vi "UTILITY Read Config File.vi"(8 "Error In":errorcluster, 10 "Main Washer Display In":T1={"Appliance Details"={"FileVersionInfo"={"FileVersion"="", "ProductName"="", "InternalName"="", "CompanyName"="", "LegalCopyright"="", "FileDescription"=""}, "Dishwasher Info"={"Open Cup Weight (gm):"=0.0, "Auto Cup Weight (gm):"=0.0, "Detergent-Dish:"="", "Inlet Temperature-Dish:"="", "Cycle Mode-Dish:"="", "Unit Control-Dish:"="", "Manufacturer-Dish:"=""}, "Washer Info"={"Hot Water Temperature (Fahrenheit):"="", "Cold Water Temperature (Fahrenheit):"="", "Capacity (cu.ft):"=0.0, "Initial Cloth Weight:"=0.0, "Cloth Lot:"=0, "Model Family:"="", "Program Name:"="", "Cycle Selection:"="", "Wash Temperature:"="", "Rinse Temperature:"="", "Load Size:"=""}, "File Name Output Array"=[], "Calibration Output Array"=[], "Appliance Common"={"Engineer:"="", "Model Number:"="", "Serial Number:"="", "Comments:"="", "Station ID:"="", "Technician:"="", "TR Number:"="", "Lab ID:"="", "Voltage:"="", "Water Pressure (PSI):"="", "Test Date:"="", "Computer Name:"="", "IP Address:"="", "Ambient RH:"="", "Frequency:"="", "Build:"="", "Filename:"="", "Test Type:"="", "Load Run #:"=0, "Ambient Temperature (F):"="", "File Path:"=path "", "Cycles Per Year"=0}, "Water Heater"={"Heating Mode:"=""}, "Dryer"={"Heat Setting:"="", "Washer Water Temperature (60 ± 5°F):"=0, "Water Hardness (PPM):"=0, "Dryness Setting:"="", "Dryer Type:"="", "Exhaust:"="", "Drying Cycle:"="", "Load Type:"="", "Nominal Load Weight"="", "Dryer Initial IMC Data"={"Measured IMC (lbs)"=0.0, "Actual Initial RMC (%)"=0.0, "RMC (Desired %)"=0.0, "Bone Dry Wt(lbs)"=0.0, "Tolerance(%)"=0.0, "Actual Final RMC (%)"=0.0, "CEF (lbf/kWh)"=0.0, "Minimum Weight (lbf)"=0.0, "Average Weight (lbf)"=0.0, "Maximum Weight (lbf)"=0.0, "Measured IMC In Range?"=FALSE, "Moisture Reduction Factor"=55.5, "Field Use Factor"=1.04, "Empty Dryer Cold Weigth"=0.0, "Energy Standard"=enum."D2-Automatic Dryer", "Weight Cloth (lbs)"=0.0, "Relative Moisture Content (%)"=0.0, "Relative Moisture Content - Avg (%)"=0.0}}}, "Display Data (RLT)"={"Status Color"=0, "Serial Number Display"="", "Cycle Count Display"=0, "Station Label Display"="", "Current Run Start Time Display"=0.0, "Board ID Display"="", "RPM Display"=0, "Current Display"=0.0, "Current Path Display"=path "", "Saving Display"=FALSE, "Unit Type Display"=enum."", "Total Time On Display"=0.0, "UI Button"=FALSE}} {"Display Data (RLT)"."Current Display" format="%.2f"; "Display Data (RLT)"."Cycle Count Display" format="%04d"; "Appliance Details"."Dryer"."Dryer Initial IMC Data"."Maximum Weight (lbf)" format="%03_6g"; "Appliance Details"."Dryer"."Dryer Initial IMC Data"."Average Weight (lbf)" format="%03_6g"; "Appliance Details"."Dryer"."Dryer Initial IMC Data"."Minimum Weight (lbf)" format="%03_6g"; "Appliance Details"."Dryer"."Dryer Initial IMC Data"."CEF (lbf/kWh)" format="%03_6g"; "Appliance Details"."Dryer"."Dryer Initial IMC Data"."Actual Final RMC (%)" format="%03_6g"; "Appliance Details"."Dryer"."Dryer Initial IMC Data"."Tolerance(%)" format="%0#_6g"; "Appliance Details"."Dryer"."Dryer Initial IMC Data"."Bone Dry Wt(lbs)" format="%03_6g"; "Appliance Details"."Dryer"."Dryer Initial IMC Data"."RMC (Desired %)" format="%0#_6g"; "Appliance Details"."Dryer"."Dryer Initial IMC Data"."Actual Initial RMC (%)" format="%03_6g"; "Appliance Details"."Dryer"."Dryer Initial IMC Data"."Measured IMC (lbs)" format="%0#_6g"}, 11 "File Locations In":T10) -> (0 "Error Out":errorcluster, 1 "GEA Information Out":T12={"GEA Diagnostic Data - Washer"={"Speed (RPM)"=0, "Load Size"=0, "Temperature"=0, "Water Pressure"=0.0, "Detergent"=0, "Fabric Softener"=0, "Tub Direction"="", "Detergent Valve"=FALSE, "Fabric Softener Valve"=FALSE, "Recirculating Pump"=FALSE, "Drain Valve"=FALSE, "Hot Valve"=FALSE, "Cold Valve"=FALSE, "Lid Closed Status"="", "Lid Lock Status"="", "Error Count"=0, "IGBT Temperature (Deg C)"=0, "Motor Speed"=0, "Latched OOB"=0, "Raw OOB"=0, "Plaster Status"=0, "Inverter Power (W)"=0, "Target Speed(BRPM)"=0, "Latched Agitate Motor Temp (Deg C)"=0, "Current Motor Temp (Deg C)"=0, "Profiler Status"="", "Current Inverter Action"="", "Error Codes"="", "Lid Locked"=FALSE, "Lid Closed"=FALSE, "9E Diagnostic Data"={"Total Cycle Time (Min)"=0, "Total Cycle Count (Current)"=0, "Total Error Count"=0, "Machine Error History"=0, "Washer UI History"=0, "Inverter Error History"=0, "Cycle Storage Limit"=0, "Error Storage Limit"=0, "Cycle Pages Supported"=0, "Error Pages Supported"=0, "Inverter Reset Count"=0}, "9F Diagnostic Data"={"Cycle Buffer Index"="", "Page Number"="", "Total Cycle Count"=0, "Delay Start Time"=0, "Stain Selected"="", "Selected Cycle"=0, "eWash"="", "Soil Level"="", "Temperature"="", "Overnight Ready"="", "Spin Setting"="", "Control Lock Status"="", "Stain Remover"="", "Steam Assist"="", "My Cycle"="", "PreWash"="", "Debug Log Enabled"="", "Rinse"="", "Signal Level"="", "PreSoak"=""}}, "Software Version"={"Critical Major SW Version"="", "Critical Minor SW Version"="", "Major SW Version"="", "Minor SW Version"="", "Parametric Data Ver. Major"="", "Parametric Data Ver. Minor"="", "Diagnostics Data Ver. Major"="", "Diagnostics Data Ver. Minor"="", "Current Personality Setting"=""}, "Debug Search Parameters"={"Pause"=["MchStdby", "MchPz", "MchIdl", "Machine Standby", "Machine Pause", "Machine Idle"], "Run"=["MchRn", "Machine Run", "Resume Process"], "EOC"=["EOC"], "Error Codes"=["Error1", "try", "rty", "inverr"]}, "Message Count"=0, "Number of Messages"=0, "Partial Message String"="", "Full Message to Save"="", "Board ID"="", "Board Index"=0, "Source Address"=0, "Destination Address"=0, "Data to send"=[], "ReceivedData"=[], "Debug/GEA Data"=[], "Command"=0, "GEA2 Reference Out"=refnum, "GEA2 Event Registration"=refnum, "Bus Data"="", "GEA Data"=[], "Network Variable Location"=0, "Water Heater GEA2 Data"={"GEA2 Label Array"=[], "PID_PARAMETERS"=[], "SUPPORTED_MODES"=[], "Button Status"={"Switch 1"=FALSE, "Switch 2"=FALSE, "Switch 3"=FALSE, "Switch 4"=FALSE, "Switch 5"=FALSE, "Switch 6"=FALSE, "Switch 7"=FALSE, "Switch 8"=FALSE, "Switch 9"=FALSE, "Switch 10"=FALSE, "Switch 11"=FALSE, "Switch 12"=FALSE, "Switch 13"=FALSE, "Switch 14"=FALSE, "Switch 15"=FALSE, "Switch 16"=FALSE}, "Status Query"={"Days Remaining (For Std Electric and Vacation)"=0, "Unit Status"="", "Current Tank Temp in Deg F"=0, "Current Setpoint in Deg F"=0, "Filter Status (% used)"=0, "Fallback Status (Fallback heating mode)"="", "Fallback Temp"=0, "\"Set Mode\" Selection"=""}, "Service Error Codes"={"Reserved"=FALSE, "Reserved 1"=FALSE, "Reserved 2"=FALSE, "Reserved 3"=FALSE, "Reserved 4"=FALSE, "Reserved 5"=FALSE, "Reserved 6"=FALSE, "Reserved 7"=FALSE, "DataFlash Fail Status"=FALSE, "Stuck Key Fail Status"=FALSE, "Dry Tank Fail Status"=FALSE, "Miswire Fail Status"=FALSE, "Reserved 8"=FALSE, "Reserved 9"=FALSE, "Reserved 10"=FALSE, "Reserved 11"=FALSE, "UE Fail Status"=FALSE, "LE Fail Status"=FALSE, "Filter Fail Status"=FALSE, "T3A Fail Status"=FALSE, "T3B Fail Status"=FALSE, "T4 Fail Status"=FALSE, "T5 Fail Status"=FALSE, "T2 Fail Status"=FALSE, "SS Cond A Status"=FALSE, "SS Cond B Status"=FALSE, "SS Cond C Status"=FALSE, "SS Cond D Status"=FALSE, "SS Cond E Status"=FALSE, "SS Cond F Status"=FALSE, "SS Fan Status"=FALSE, "CMP Fail Status"=FALSE}, "HEM_KWH_DATA"=[], "OTHER_FAULT_COUNTS"=[], "GEA2 Raw Message"="", "Hyperterminal Data"={"Source"=0, "Destination"=0, "Command"=0, "Length"=0, "CRC"=0, "UE - state (1/0 on off)"=0, "LE - state (1/0 on off)"=0, "Comp - state (1/0 on off)"=0, "Fan  - state (1/0 on off)"=0, "Setpoint Deg F"=0, "T2(TankSensor)"=0.0, "T3A(EvapIn)"=0.0, "T3B(EvapOut)"=0.0, "T4(CompressorDischarge)"=0.0, "T5(Ambient)"=0.0, "Current"=0.0, "Voltage (Volts)"=0, "EEV Position (0-480)"=0, "Reason for last heating cycle termination"=0, "Reason Data word 1"="", "Reason Data word 2"="", "Reason Data word 3"="", "Reason Data word 4"="", "SW Debug Data"="", "Flow Events (Bit Encoded)"=0, "Heating Control Mode"=0}, "Extra Data"={"Water Capacity (Gallons)"=0, "Max Vacation Duration Days"=0, "Min Vacation Duration Days"=0, "Max Set Point (Deg F)"=0, "Min Set Point (Deg F)"=0, "T5 Resistance"=0, "T4 Resistance"=0, "T3B Resistance"=0, "T2 Resistance"=0, "STD_ELEC_RANGE"="", "SS_FAULT_COUNTS"="", "SERIAL_NUMBER"="", "READ_PERSONALITY"=0, "RQST_OVERRIDE_STATUS"="", "MODEL_SELECT_AD_VALUE"=0, "MODEL NUMBER"="", "IDLB_RESISTANCE"=0, "DSM Override Status"="", "RQST_DATA_FROM_Memory"="", "RQST_DATA_FROM_DATA_FLASH"="", "RQST_CURRENT_PID_SH_TARGET"=0, "Unit System Mode"=""}}} {"Water Heater GEA2 Data"."Hyperterminal Data"."CRC" format="%x"; "Water Heater GEA2 Data"."Hyperterminal Data"."Length" format="%x"; "Water Heater GEA2 Data"."Hyperterminal Data"."Command" format="%x"; "Water Heater GEA2 Data"."Hyperterminal Data"."Destination" format="%x"; "Water Heater GEA2 Data"."Hyperterminal Data"."Source" format="%x"; "Destination Address" format="%x"; "Source Address" format="%x"; "Command" format="%.0x"; "Data to send" format="%x"; "ReceivedData" format="%x"}, 2 "Main Washer Display Out":T1={"Appliance Details"={"FileVersionInfo"={"FileVersion"="", "ProductName"="", "InternalName"="", "CompanyName"="", "LegalCopyright"="", "FileDescription"=""}, "Dishwasher Info"={"Open Cup Weight (gm):"=0.0, "Auto Cup Weight (gm):"=0.0, "Detergent-Dish:"="", "Inlet Temperature-Dish:"="", "Cycle Mode-Dish:"="", "Unit Control-Dish:"="", "Manufacturer-Dish:"=""}, "Washer Info"={"Hot Water Temperature (Fahrenheit):"="", "Cold Water Temperature (Fahrenheit):"="", "Capacity (cu.ft):"=0.0, "Initial Cloth Weight:"=0.0, "Cloth Lot:"=0, "Model Family:"="", "Program Name:"="", "Cycle Selection:"="", "Wash Temperature:"="", "Rinse Temperature:"="", "Load Size:"=""}, "File Name Output Array"=[], "Calibration Output Array"=[], "Appliance Common"={"Engineer:"="", "Model Number:"="", "Serial Number:"="", "Comments:"="", "Station ID:"="", "Technician:"="", "TR Number:"="", "Lab ID:"="", "Voltage:"="", "Water Pressure (PSI):"="", "Test Date:"="", "Computer Name:"="", "IP Address:"="", "Ambient RH:"="", "Frequency:"="", "Build:"="", "Filename:"="", "Test Type:"="", "Load Run #:"=0, "Ambient Temperature (F):"="", "File Path:"=path "", "Cycles Per Year"=60}, "Water Heater"={"Heating Mode:"=""}, "Dryer"={"Heat Setting:"="", "Washer Water Temperature (60 ± 5°F):"=60, "Water Hardness (PPM):"=17, "Dryness Setting:"="", "Dryer Type:"="", "Exhaust:"="", "Drying Cycle:"="", "Load Type:"="", "Nominal Load Weight"="", "Dryer Initial IMC Data"={"Measured IMC (lbs)"=7.0, "Actual Initial RMC (%)"=7.0, "RMC (Desired %)"=100.0, "Bone Dry Wt(lbs)"=7.0, "Tolerance(%)"=5.0, "Actual Final RMC (%)"=0.0, "CEF (lbf/kWh)"=0.0, "Minimum Weight (lbf)"=0.0, "Average Weight (lbf)"=0.0, "Maximum Weight (lbf)"=0.0, "Measured IMC In Range?"=FALSE, "Moisture Reduction Factor"=55.5, "Field Use Factor"=1.04, "Empty Dryer Cold Weigth"=0.0, "Energy Standard"=enum."D2-Automatic Dryer", "Weight Cloth (lbs)"=0.0, "Relative Moisture Content (%)"=0.0, "Relative Moisture Content - Avg (%)"=0.0}}}, "Display Data (RLT)"={"Status Color"=0, "Serial Number Display"="", "Cycle Count Display"=0, "Station Label Display"="", "Current Run Start Time Display"=0.0, "Board ID Display"="", "RPM Display"=0, "Current Display"=0.0, "Current Path Display"=path "", "Saving Display"=FALSE, "Unit Type Display"=enum."", "Total Time On Display"=0.0, "UI Button"=FALSE}} {"Display Data (RLT)"."Current Display" format="%.2f"; "Display Data (RLT)"."Cycle Count Display" format="%04d"; "Appliance Details"."Dryer"."Dryer Initial IMC Data"."Maximum Weight (lbf)" format="%03_6g"; "Appliance Details"."Dryer"."Dryer Initial IMC Data"."Average Weight (lbf)" format="%03_6g"; "Appliance Details"."Dryer"."Dryer Initial IMC Data"."Minimum Weight (lbf)" format="%03_6g"; "Appliance Details"."Dryer"."Dryer Initial IMC Data"."CEF (lbf/kWh)" format="%03_6g"; "Appliance Details"."Dryer"."Dryer Initial IMC Data"."Actual Final RMC (%)" format="%03_6g"; "Appliance Details"."Dryer"."Dryer Initial IMC Data"."Tolerance(%)" format="%0#_6g"; "Appliance Details"."Dryer"."Dryer Initial IMC Data"."Bone Dry Wt(lbs)" format="%03_6g"; "Appliance Details"."Dryer"."Dryer Initial IMC Data"."RMC (Desired %)" format="%0#_6g"; "Appliance Details"."Dryer"."Dryer Initial IMC Data"."Actual Initial RMC (%)" format="%03_6g"; "Appliance Details"."Dryer"."Dryer Initial IMC Data"."Measured IMC (lbs)" format="%0#_6g"})   [LabVIEW 2018]
uses:
  Washer HCC/Washer HCC NEWFI/Type Definitions/ViperHawk/ViperHawk Data.ctl
  Washer HCC/Washer HCC NEWFI/Type Definitions/ViperHawk/ViperHawk Diagnostic Data.ctl
  Save File/Public/Type Definitions/Save File Software Version.ctl
  Washer HCC/Washer HCC NEWFI/Type Definitions/ViperHawk/ViperHawk Search Control.ctl
  C:/Andrew_Treasure_Chest/NI-2010/Trunk/Utility/LabVIEW GEA2 Toolkit v1.0.0.0/Appliance.NET/GeaCommunication.dll
  LabVIEW GEA2 Toolkit v1.0.0.0/Appliance.NET/GeaCommunication.dll
  LabVIEW GEA2 Toolkit v1.0.0.0/type defs/Data Out.ctl
  GEA2 Commands/HEWH/Type Definitions/GEA2 Commands WaterHeater GEA2 Data.ctl
  GEA2 Commands/HEWH/Type Definitions/GEA2 Commands Button Status.ctl
  GEA2 Commands/HEWH/Type Definitions/GEA2 Commands Status Query.ctl
  GEA2 Commands/HEWH/Type Definitions/GEA2 Commands Service Error Codes.ctl
  Save File/Public/Type Definitions/Save File Washer.ctl
  Save File/File Setup (Public)/Type Definition/Save File DISH Dishwasher Details.ctl
  <vilib>/Platform/fileVersionInfo.llb/FileVersionInformation.ctl
  Washer DOE/Type Definitions/DOE Appliance Common.ctl
  Custom Pallet Controls/Custom Pallet String.ctl
  Save File/File Setup (Public)/Type Definition/DPT IMC Data.ctl
  Washer DOE/Type Definitions/DOE Dryer Standard.ctl
  Save File/Public/Type Definitions/Save File Appliance Display.ctl
  Save File/Public/Type Definitions/Save File Unit Type.ctl
  Save File/File Setup (Public)/Type Definition/Save File DOE File Path Control.ctl
  Save File/File Setup (Public)/Type Definition/Save File DOE Data Save Filepaths.ctl
  LabVIEW GEA2 Toolkit v1.0.0.0/library/GEA2_Toolkit.lvlib
  Save File/Save File.lvlib
  Save File/File Setup.lvlib
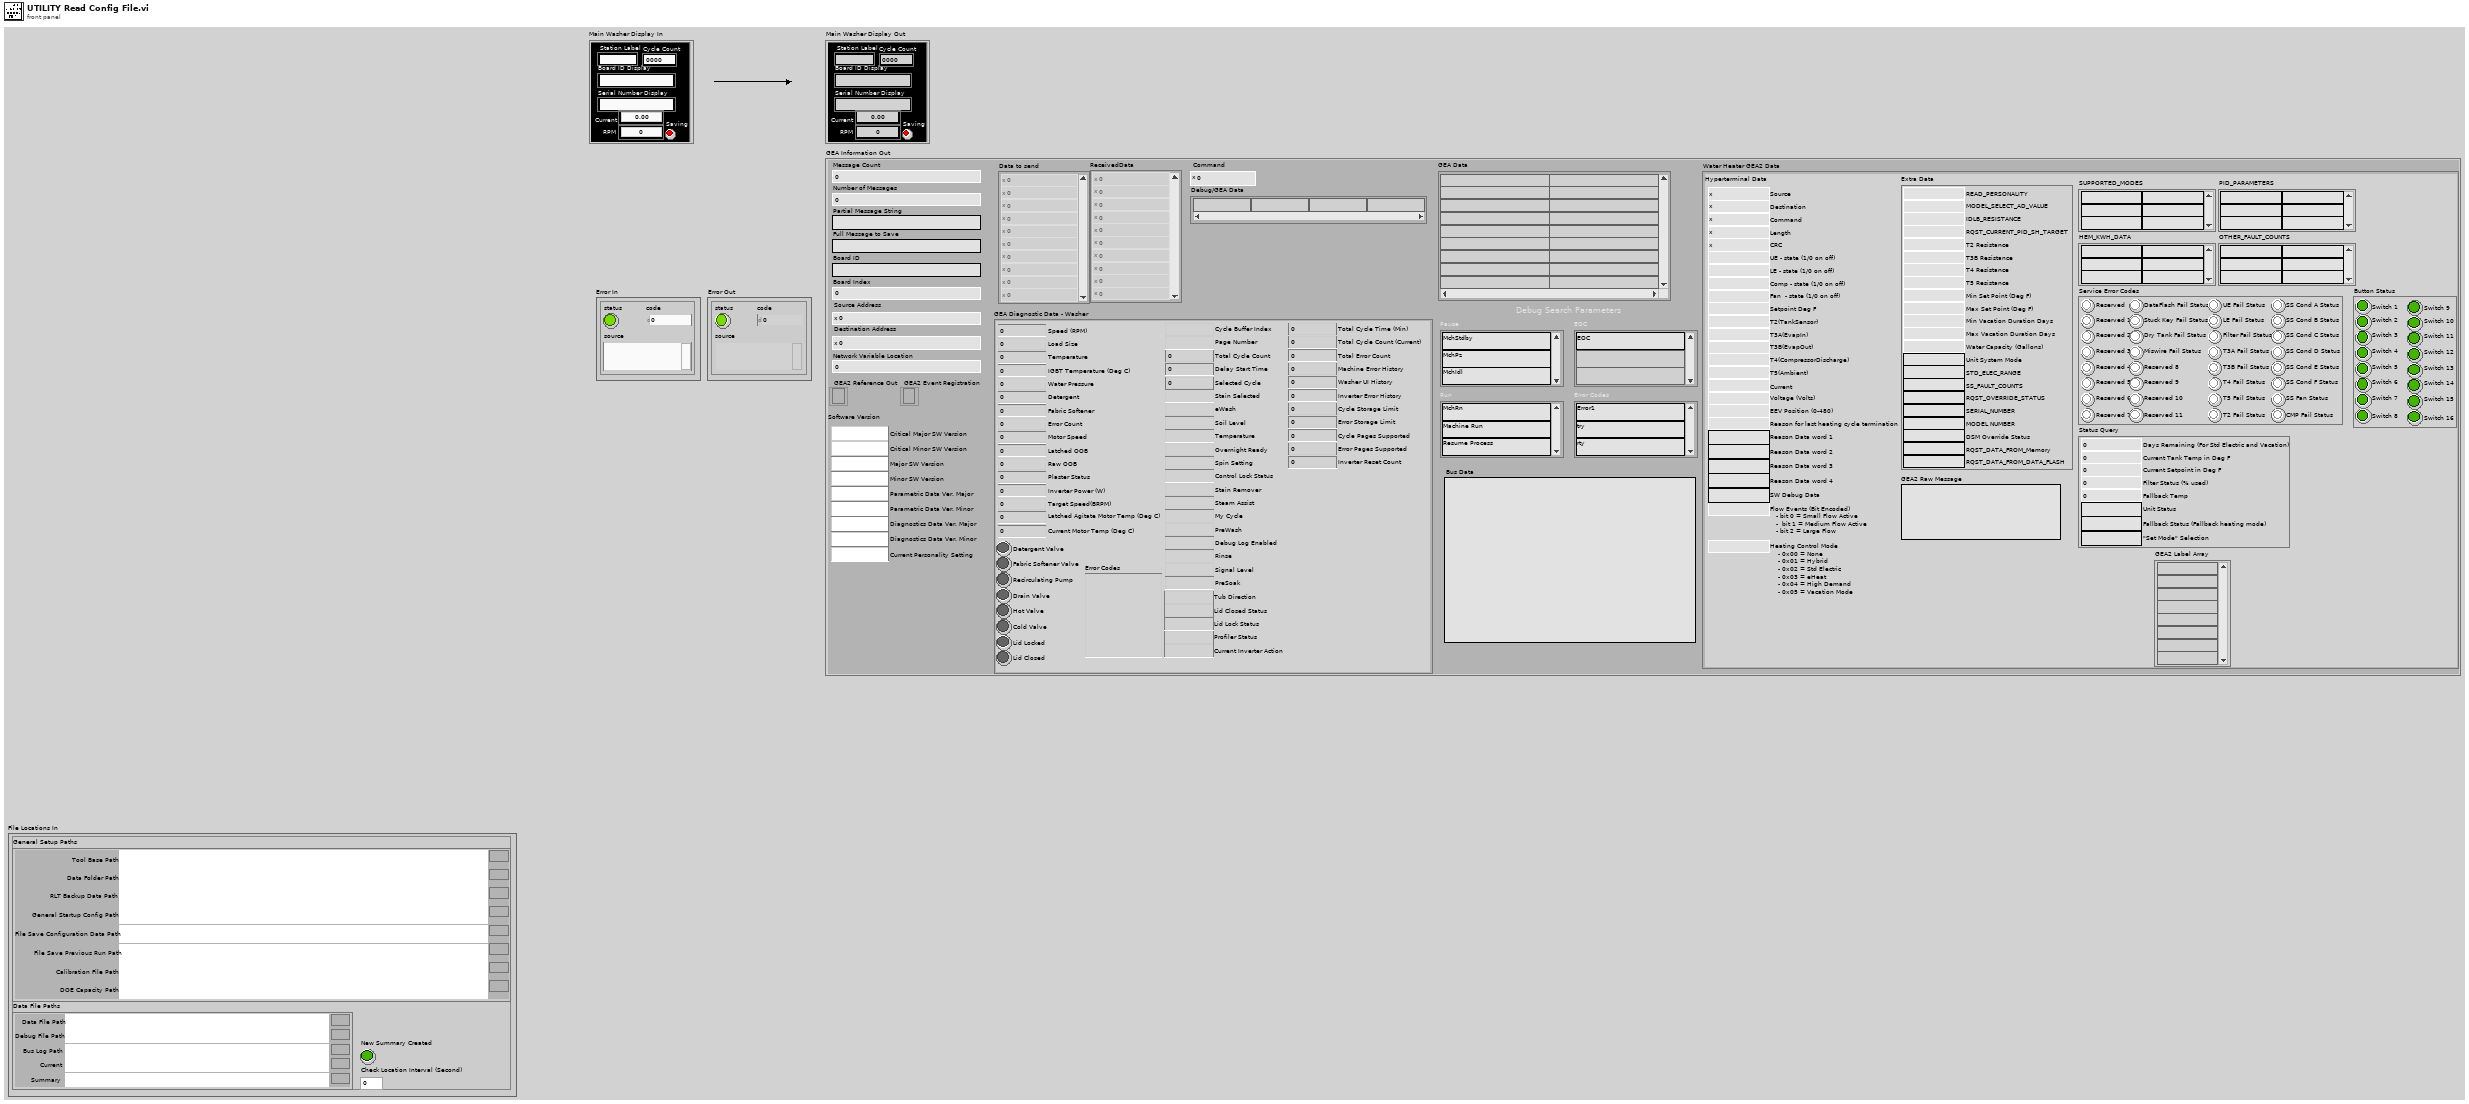
[diagram p1: front panel]
types:
  T1 = typedef "Save File.lvlib/Save File Washer.ctl" = cluster{"Appliance Details":T2, "Display Data (RLT)":T8}
  T2 = typedef "File Setup.lvlib/Save File DISH Dishwasher Details.ctl" = cluster{"FileVersionInfo":T3, "Dishwasher Info":cluster{"Open Cup Weight (gm):":dbl, "Auto Cup Weight (gm):":dbl, "Detergent-Dish:":string, "Inlet Temperature-Dish:":string, "Cycle Mode-Dish:":string, "Unit Control-Dish:":string, "Manufacturer-Dish:":string}, "Washer Info":cluster{"Hot Water Temperature (Fahrenheit):":string, "Cold Water Temperature (Fahrenheit):":string, "Capacity (cu.ft):":dbl, "Initial Cloth Weight:":dbl, "Cloth Lot:":i32, "Model Family:":string, "Program Name:":string, "Cycle Selection:":string, "Wash Temperature:":string, "Rinse Temperature:":string, "Load Size:":string}, "File Name Output Array":string[][], "Calibration Output Array":string[][], "Appliance Common":T4, "Water Heater":cluster{"Heating Mode:":string}, "Dryer":cluster{"Heat Setting:":T5, "Washer Water Temperature (60 ± 5°F):":u16, "Water Hardness (PPM):":u16, "Dryness Setting:":T5, "Dryer Type:":string, "Exhaust:":string, "Drying Cycle:":string, "Load Type:":string, "Nominal Load Weight":string, "Dryer Initial IMC Data":T6}}
  T3 = typedef "FileVersionInformation.ctl" = cluster{"FileVersion":string, "ProductName":string, "InternalName":string, "CompanyName":string, "LegalCopyright":string, "FileDescription":string}
  T4 = typedef "DOE Appliance Common.ctl" = cluster{"Engineer:":string, "Model Number:":string, "Serial Number:":string, "Comments:":string, "Station ID:":string, "Technician:":string, "TR Number:":string, "Lab ID:":string, "Voltage:":string, "Water Pressure (PSI):":string, "Test Date:":string, "Computer Name:":string, "IP Address:":string, "Ambient RH:":string, "Frequency:":string, "Build:":string, "Filename:":string, "Test Type:":string, "Load Run #:":i32, "Ambient Temperature (F):":string, "File Path:":path, "Cycles Per Year":u32}
  T5 = typedef "Custom Pallet String.ctl" = string
  T6 = typedef "DPT IMC Data.ctl" = cluster{"Measured IMC (lbs)":dbl, "Actual Initial RMC (%)":dbl, "RMC (Desired %)":dbl, "Bone Dry Wt(lbs)":dbl, "Tolerance(%)":dbl, "Actual Final RMC (%)":dbl, "CEF (lbf/kWh)":dbl, "Minimum Weight (lbf)":dbl, "Average Weight (lbf)":dbl, "Maximum Weight (lbf)":dbl, "Measured IMC In Range?":bool, "Moisture Reduction Factor":dbl, "Field Use Factor":dbl, "Empty Dryer Cold Weigth":dbl, "Energy Standard":T7, "Weight Cloth (lbs)":dbl, "Relative Moisture Content (%)":dbl, "Relative Moisture Content - Avg (%)":dbl}
  T7 = typedef "DOE Dryer Standard.ctl" = enum16{"D2-Automatic Dryer", "D2-Timer Dryer", "D1-Automatic Dryer", "D1-Timer Dryer", "Other"}
  T8 = typedef "Save File Appliance Display.ctl" = cluster{"Status Color":u32, "Serial Number Display":string, "Cycle Count Display":i32, "Station Label Display":string, "Current Run Start Time Display":dbl, "Board ID Display":string, "RPM Display":u32, "Current Display":dbl, "Current Path Display":path, "Saving Display":bool, "Unit Type Display":T9, "Total Time On Display":dbl, "UI Button":bool}
  T9 = typedef "Save File.lvlib/Save File Unit Type.ctl" = enum32{"", "Viper", "Hawk", "2015"}
  T10 = typedef "File Setup.lvlib/Save File DOE File Path Control.ctl" = cluster{"General Setup Paths":cluster{"Calibration File Path":path, "DOE Capacity Path":path, "Data Folder Path":path, "RLT Backup Data Path":path, "Tool Base Path":path, "General Startup Config Path":path, "File Save Previous Run Path":path, "File Save Configuration Data Path":path}, "Data File Paths":T11, "New Summary Created":bool, "Check Location Interval (Second)":i32}
  T11 = typedef "File Setup.lvlib/Save File DOE Data Save Filepaths.ctl" = cluster{"Data File Path":path, "Debug File Path":path, "Bus Log Path":path, "Current":path, "Summary":path}
  T12 = typedef "ViperHawk Data.ctl" = cluster{"GEA Diagnostic Data - Washer":T13, "Software Version":T14, "Debug Search Parameters":T15, "Message Count":i32, "Number of Messages":i32, "Partial Message String":string, "Full Message to Save":string, "Board ID":string, "Board Index":i32, "Source Address":u8, "Destination Address":u8, "Data to send":u8[], "ReceivedData":u8[], "Debug/GEA Data":string[], "Command":u8, "GEA2 Reference Out":refnum<k24>, "GEA2 Event Registration":refnum<event-registration>, "Bus Data":string, "GEA Data":string[][], "Network Variable Location":i32, "Water Heater GEA2 Data":T16}
  T13 = typedef "ViperHawk Diagnostic Data.ctl" = cluster{"Speed (RPM)":u32, "Load Size":u32, "Temperature":u32, "Water Pressure":dbl, "Detergent":u32, "Fabric Softener":u32, "Tub Direction":string, "Detergent Valve":bool, "Fabric Softener Valve":bool, "Recirculating Pump":bool, "Drain Valve":bool, "Hot Valve":bool, "Cold Valve":bool, "Lid Closed Status":string, "Lid Lock Status":string, "Error Count":u32, "IGBT Temperature (Deg C)":u32, "Motor Speed":u32, "Latched OOB":u32, "Raw OOB":u32, "Plaster Status":u32, "Inverter Power (W)":u32, "Target Speed(BRPM)":u32, "Latched Agitate Motor Temp (Deg C)":u32, "Current Motor Temp (Deg C)":u32, "Profiler Status":string, "Current Inverter Action":string, "Error Codes":string, "Lid Locked":bool, "Lid Closed":bool, "9E Diagnostic Data":cluster{"Total Cycle Time (Min)":u32, "Total Cycle Count (Current)":u16, "Total Error Count":u16, "Machine Error History":u32, "Washer UI History":u32, "Inverter Error History":u32, "Cycle Storage Limit":u8, "Error Storage Limit":u8, "Cycle Pages Supported":u8, "Error Pages Supported":u8, "Inverter Reset Count":u16}, "9F Diagnostic Data":cluster{"Cycle Buffer Index":string, "Page Number":string, "Total Cycle Count":u32, "Delay Start Time":u32, "Stain Selected":string, "Selected Cycle":u32, "eWash":string, "Soil Level":string, "Temperature":string, "Overnight Ready":string, "Spin Setting":string, "Control Lock Status":string, "Stain Remover":string, "Steam Assist":string, "My Cycle":string, "PreWash":string, "Debug Log Enabled":string, "Rinse":string, "Signal Level":string, "PreSoak":string}}
  T14 = typedef "Save File.lvlib/Save File Software Version.ctl" = cluster{"Critical Major SW Version":string, "Critical Minor SW Version":string, "Major SW Version":string, "Minor SW Version":string, "Parametric Data Ver. Major":string, "Parametric Data Ver. Minor":string, "Diagnostics Data Ver. Major":string, "Diagnostics Data Ver. Minor":string, "Current Personality Setting":string}
  T15 = typedef "ViperHawk Search Control.ctl" = cluster{"Pause":string[], "Run":string[], "EOC":string[], "Error Codes":string[]}
  T16 = typedef "GEA2 Commands WaterHeater GEA2 Data.ctl" = cluster{"GEA2 Label Array":string[], "PID_PARAMETERS":string[][], "SUPPORTED_MODES":string[][], "Button Status":T17, "Status Query":T18, "Service Error Codes":T19, "HEM_KWH_DATA":string[][], "OTHER_FAULT_COUNTS":string[][], "GEA2 Raw Message":string, "Hyperterminal Data":cluster{"Source":u8, "Destination":u8, "Command":u8, "Length":u8, "CRC":u16, "UE - state (1/0 on off)":u8, "LE - state (1/0 on off)":u8, "Comp - state (1/0 on off)":u8, "Fan  - state (1/0 on off)":u8, "Setpoint Deg F":i32, "T2(TankSensor)":dbl, "T3A(EvapIn)":dbl, "T3B(EvapOut)":dbl, "T4(CompressorDischarge)":dbl, "T5(Ambient)":dbl, "Current":dbl, "Voltage (Volts)":u16, "EEV Position (0-480)":u16, "Reason for last heating cycle termination":u16, "Reason Data word 1":string, "Reason Data word 2":string, "Reason Data word 3":string, "Reason Data word 4":string, "SW Debug Data":string, "Flow Events (Bit Encoded)":u16, "Heating Control Mode":u16}, "Extra Data":cluster{"Water Capacity (Gallons)":u32, "Max Vacation Duration Days":u32, "Min Vacation Duration Days":u32, "Max Set Point (Deg F)":u32, "Min Set Point (Deg F)":u32, "T5 Resistance":u32, "T4 Resistance":u32, "T3B Resistance":u32, "T2 Resistance":u32, "STD_ELEC_RANGE":string, "SS_FAULT_COUNTS":string, "SERIAL_NUMBER":string, "READ_PERSONALITY":u8, "RQST_OVERRIDE_STATUS":string, "MODEL_SELECT_AD_VALUE":u32, "MODEL NUMBER":string, "IDLB_RESISTANCE":u32, "DSM Override Status":string, "RQST_DATA_FROM_Memory":string, "RQST_DATA_FROM_DATA_FLASH":string, "RQST_CURRENT_PID_SH_TARGET":u16, "Unit System Mode":string}}
  T17 = typedef "GEA2 Commands Button Status.ctl" = cluster{"Switch 1":bool, "Switch 2":bool, "Switch 3":bool, "Switch 4":bool, "Switch 5":bool, "Switch 6":bool, "Switch 7":bool, "Switch 8":bool, "Switch 9":bool, "Switch 10":bool, "Switch 11":bool, "Switch 12":bool, "Switch 13":bool, "Switch 14":bool, "Switch 15":bool, "Switch 16":bool}
  T18 = typedef "GEA2 Commands Status Query.ctl" = cluster{"Days Remaining (For Std Electric and Vacation)":u8, "Unit Status":string, "Current Tank Temp in Deg F":u8, "Current Setpoint in Deg F":u8, "Filter Status (% used)":u8, "Fallback Status (Fallback heating mode)":string, "Fallback Temp":u8, "\"Set Mode\" Selection":string}
  T19 = typedef "GEA2 Commands Service Error Codes.ctl" = cluster{"Reserved":bool, "Reserved 1":bool, "Reserved 2":bool, "Reserved 3":bool, "Reserved 4":bool, "Reserved 5":bool, "Reserved 6":bool, "Reserved 7":bool, "DataFlash Fail Status":bool, "Stuck Key Fail Status":bool, "Dry Tank Fail Status":bool, "Miswire Fail Status":bool, "Reserved 8":bool, "Reserved 9":bool, "Reserved 10":bool, "Reserved 11":bool, "UE Fail Status":bool, "LE Fail Status":bool, "Filter Fail Status":bool, "T3A Fail Status":bool, "T3B Fail Status":bool, "T4 Fail Status":bool, "T5 Fail Status":bool, "T2 Fail Status":bool, "SS Cond A Status":bool, "SS Cond B Status":bool, "SS Cond C Status":bool, "SS Cond D Status":bool, "SS Cond E Status":bool, "SS Cond F Status":bool, "SS Fan Status":bool, "CMP Fail Status":bool}
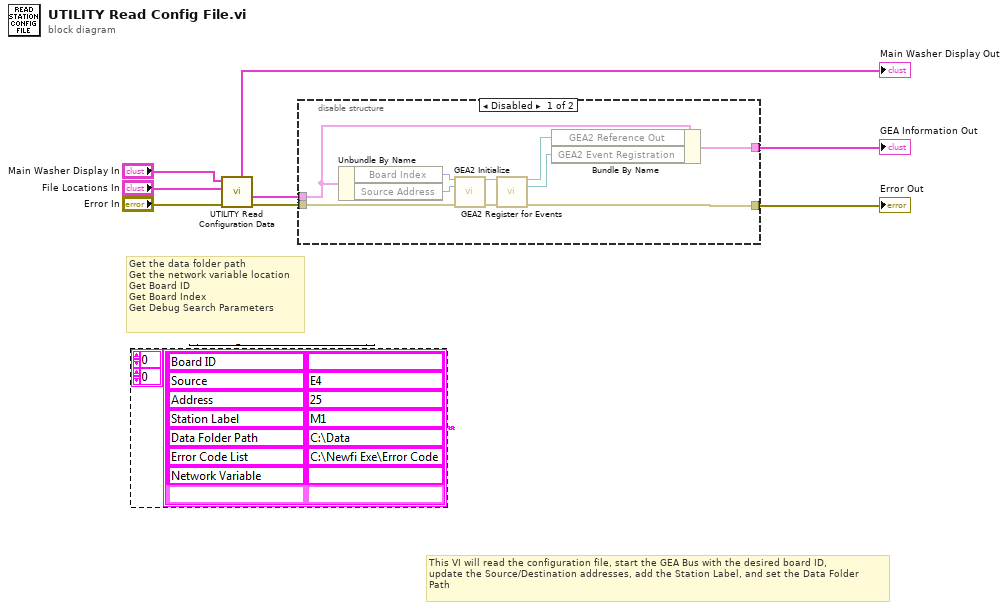
[diagram p0: block diagram]
diagram:
  # "Get the data folder path\nGet the network variable location\nGet Board ID\nGet Board Index\nGet Debug Search Parameters"
  # "This VI will read the configuration file, start the GEA Bus with the desired board ID,\nupdate the Source/Destination addresses, add the Station Label, and set the Data Folder\nPath"
  n1 = call "UTILITY Read Configuration Data.vi"("error in (no error)"="Error In", "File Locations In"="File Locations In", "Main Washer Display In"="Main Washer Display In") -> ("error out"=w3:errorcluster, "GEA Information In out"=w2:T12, "Main Washer Display Out"=→"Main Washer Display Out":T1)  [unwired: 6 in]
  n2 = disable-structure shown="Disabled" {
    disable-tunnel: [w18 _] -> w6
    disable-tunnel: [w14 _] -> w5
    disable-tunnel: w3 -> [w11 _]
    disable-tunnel: w2 -> [w10 _]
    frame Disabled {
      n3 = Unbundle By Name(w10) -> ("Board Index"=w15:i32, "Source Address"=w9:u8)
      n4 = call "GEA2 Initialize.vi"("Board Index"=w15, "Source Address"=w9, "error in"=w11) -> ("GEA2 Reference Out"=w16:refnum<k24>, "error out"=w17:errorcluster)  [unwired: 10 in, 1 out]
      n5 = call "GEA2 Register for Events.vi"("GEA2 Reference In"=w16, "Error In"=w17) -> ("GEA2 Reference Out"=w12:refnum<k24>, "GEA2 Event Registration"=w13:refnum<event-registration>, "Error Out"=w14:errorcluster)  [unwired: 11 in]
      n6 = Bundle By Name(cluster=w10, "GEA2 Reference Out"=w12, "GEA2 Event Registration"=w13) -> (w18:T12)
    }
    frame Enabled {
    }
  }
  "GEA Information Out" <- w6
  "Error Out" <- w5
